vi "Parse LVClasses by Type.vi"(10 "Type":string, 11 "Input":string) -> (3 "Relative Paths":path[](array[path]))   [LabVIEW 2020, in "Test Finder.lvclass"]
uses:
  Test Finder.lvclass
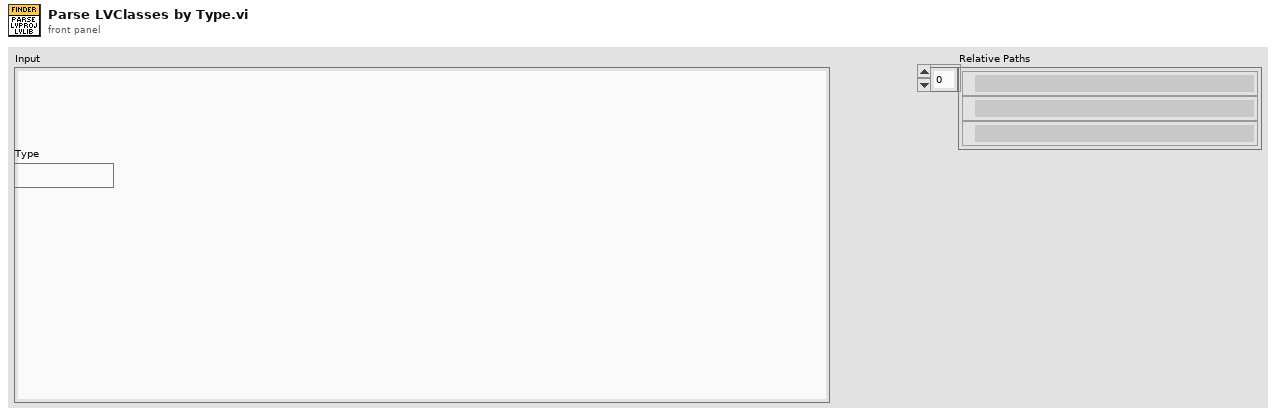
[diagram p1: front panel]
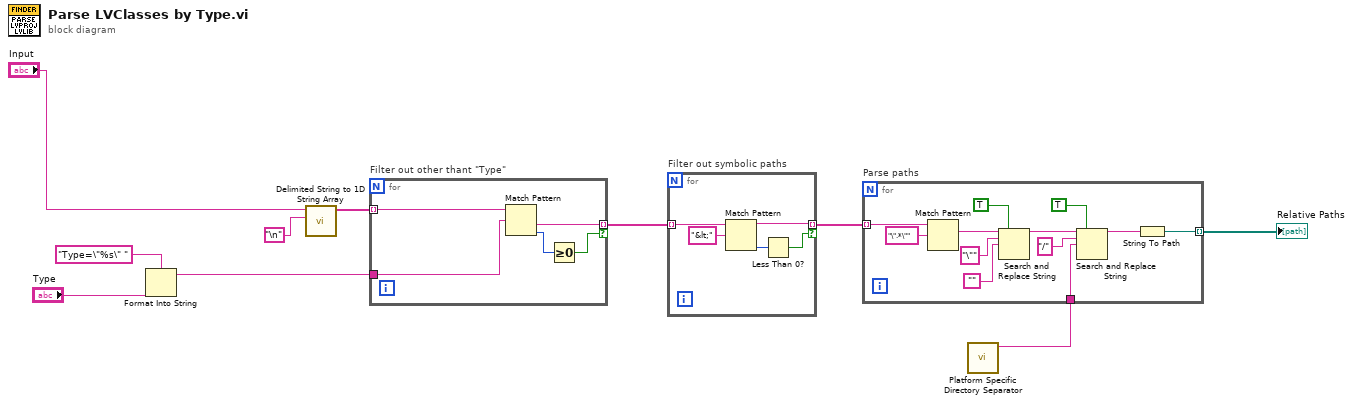
[diagram p0: block diagram]
diagram:
  n1 = Format Into String(format string="Type=\"%s\" " ("regular expression"), "Type") -> (resulting string=w5:string)  [unwired: 2 in, 1 out]
  n2 = call <vilib>:"Delimited String to 1D String Array.vi"("delimiter"="\n", "delimited string"="Input") -> ("string array"=w9:string[])  [unwired: 9 in]
  n3 = for "Filter out other thant \"Type\"" {
    tunnel: w9 -> [w15] mode=indexing
    tunnel: [w14] -> w2 mode=indexing if=w12
    tunnel: w5 -> [w11]
    n4 = Match Pattern(string=w15, regular expression=w11) -> (after substring=w14:string, offset past match=w13:i32)  [unwired: 1 in, 2 out]
    n5 = Greater Or Equal To 0?(x=w13) -> (x >= 0?=w12:bool)
  }
  n6 = for "Filter out symbolic paths" {
    tunnel: [w19] -> w3 mode=indexing if=w16
    tunnel: w2 -> [w20] mode=indexing
    n7 = Match Pattern(string=w20, regular expression="&lt;") -> (before substring=w19:string, offset past match=w17:i32)  [unwired: 1 in, 2 out]
    n8 = Less Than 0?(x=w17) -> (x < 0?=w16:bool)
  }
  n9 = call "Platform Specific Directory Separator.vi"() -> ("search string"=w1:string)  [unwired: 11 in]
  n10 = for "Parse paths" {
    tunnel: w3 -> [w32] mode=indexing
    tunnel: [w25] -> w4 mode=indexing
    tunnel: w1 -> [w21]
    n11 = Match Pattern(string=w32, regular expression="\".*\"") -> (match substring=w30:string)  [unwired: 1 in, 3 out]
    n12 = Search and Replace String(replace all?=TRUE ("replace all? (F)"), input string=w30, search string="\"", replace string="") -> (result string=w26:string)  [unwired: 4 in, 3 out]
    n13 = Search and Replace String(replace all?=TRUE ("replace all? (F)"), input string=w26, search string="/", replace string=w21) -> (result string=w24:string)  [unwired: 4 in, 3 out]
    n14 = String To Path(string=w24) -> (path=w25:path)
  }
  "Relative Paths" <- w4
